vi "Smp_RAM_transfer.vi"(0 "Connection ID":T1, 5 "SaveFilePath":path caption="Temp file path", 9 "Read point":i32=1000, 11 "error in (no error)":errorcluster) -> (3 "Error Code":i16, 4 "Connection ID Out":T1, 6 "SaveFilePath.ref":path caption="Temp file path.ref", 10 "Stop":bool, 15 "error out":errorcluster)   [LabVIEW 2017]
uses:
  Driver/ConnectionID.ctl
  GL860_Driver.lvlib
panel:
  out "Progress bar":u8(slide) max=100 scale=0.0..100.0
  in  "Stop":bool
  # "Now transferring data..."
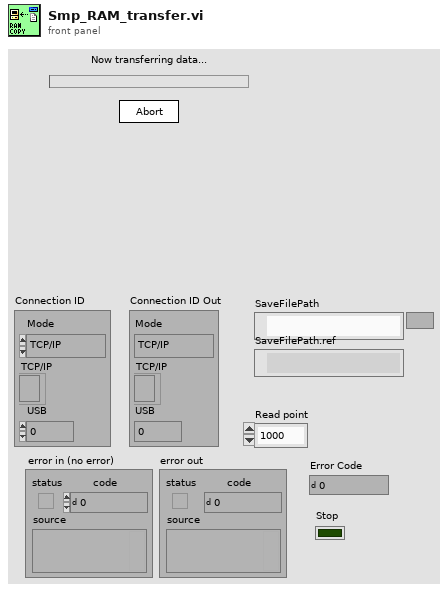
[diagram p1: front panel]
types:
  T1 = typedef "ConnectionID.ctl" = cluster{"Mode":enum16{"TCP/IP", "USB"}, "TCP/IP":refnum<k5>, "USB":i32}
  T2 = enum16{"open", "replace", "create", "open or create", "replace or create", "replace or create with confirmation"}
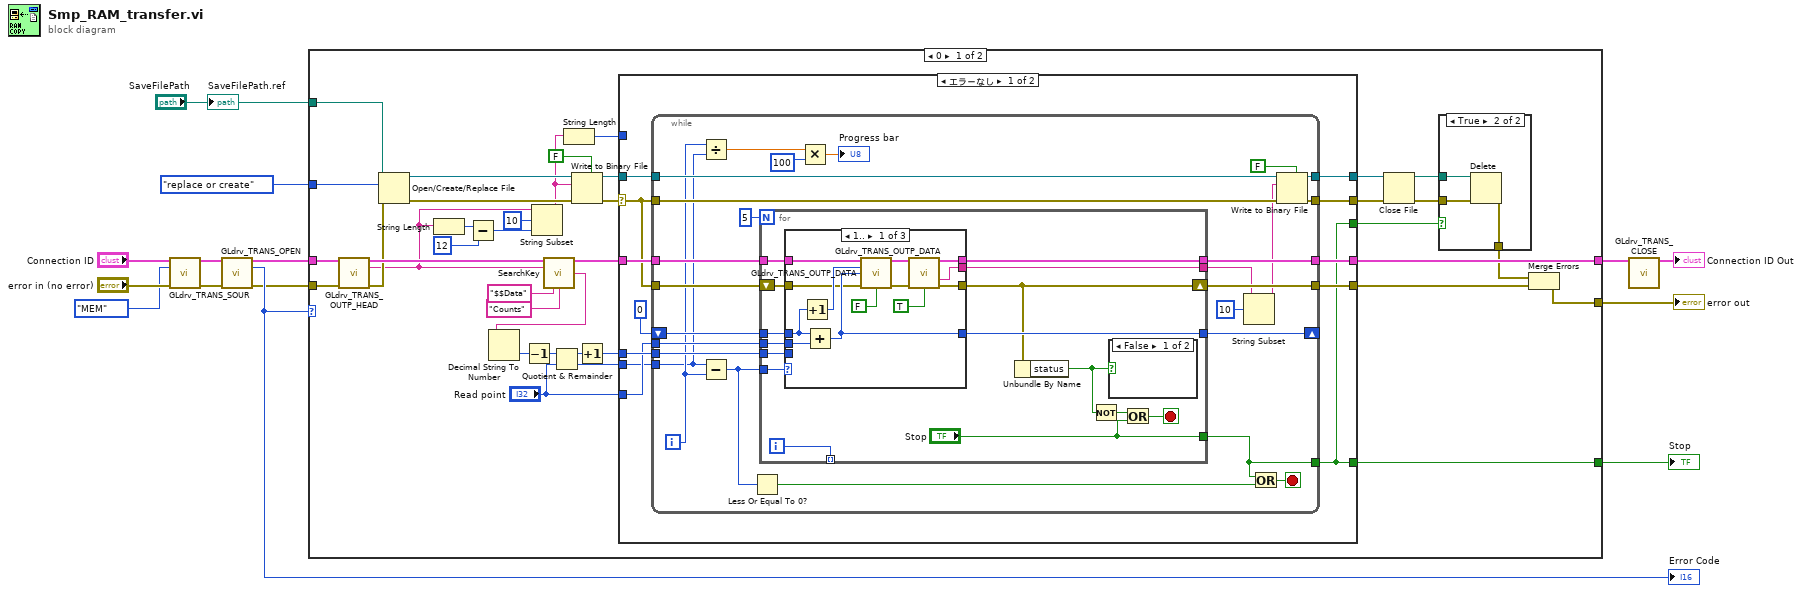
[diagram p0: block diagram]
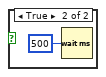
[diagram p3: hidden frame]
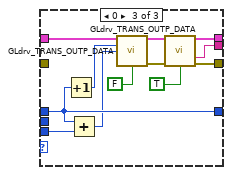
[diagram p5: hidden frame]
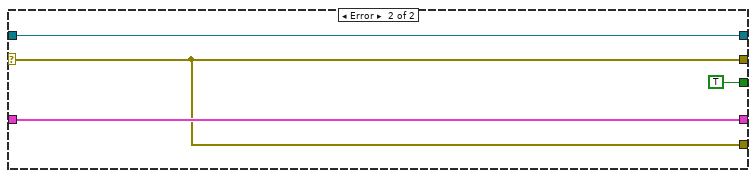
[diagram p6: hidden frame]
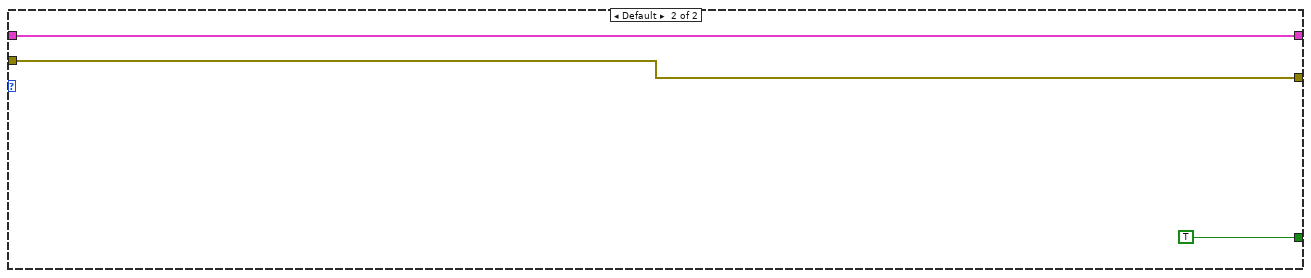
[diagram p7: hidden frame]
diagram:
  n1 = call "GLdrv_TRANS_SOUR.vi"("Connection ID"="Connection ID", "Mode"=enum16{"DISK", "MEM"}."MEM", "error in (no error)"="error in (no error)") -> ("Connection ID Out"=w8:T1, "error out"=w6:errorcluster)  [unwired: 9 in, 2 out]
  n2 = call "GLdrv_TRANS_OPEN.vi"("Connection ID"=w8, "error in (no error)"=w6) -> ("Connection ID Out"=w5:T1, "Error Code"=w7:i16, "error out"=w4:errorcluster)  [unwired: 10 in, 1 out]
  "Error Code" <- w7
  n3 = case shown="0" w7 {
    tunnel: [w50 w142] -> w3
    tunnel: [w48 w143] -> w1
    tunnel: [w43 TRUE ("Stop")] -> w14
    tunnel: "SaveFilePath" -> [w19 _]
    tunnel: T2."replace or create" ("operation (0:open)") -> [w40 _]
    tunnel: w5 -> [w39 w142]
    tunnel: w4 -> [w38 w143]
    frame 0 {
      n4 = call "GLdrv_TRANS_OUTP_HEAD.vi"("Connection ID"=w39, "error in (no error)"=w38) -> ("Connection ID Out"=w37:T1, "Data out"=w25:string, "error out"=w36:errorcluster)  [unwired: 11 in]
      n5 = Open/Create/Replace File(file path (use dialog)=w19, error in=w36, operation (0:open)=w40) -> (refnum out=w33:refnum<file>, error out=w34:errorcluster)  [unwired: 4 out]
      n6 = String Length(string=w25) -> (length=w24:i32)
      n7 = Subtract(x=w24, y=12) -> (x-y=w22:i32)
      n8 = String Subset(string=w25, offset (0)=10 ("オフセット（0）"), length (rest)=w22) -> (substring=w21:string)
      n9 = call "SearchKey.vi"("In"=w25, "KEY1"="$$Data", "KEY2"="Counts") -> ("String"=w27:string)  [unwired: 12 out]
      n10 = Decimal String To Number(string=w27) -> (number=w28:i32)  [unwired: 2 in, 1 out]
      n11 = Decrement(x=w28) -> (x-1=w42:i32)
      n12 = Quotient & Remainder(x=w42, y="Read point") -> (x-y*floor(x/y)=w45:i32, floor(x/y)=w44:i32)
      n13 = String Length(string=w21) -> (length=w20:i32)
      n14 = Write to Binary File(file (use dialog)=w33, data=w21, error in=w34, 5:FALSE ("prepend array or string size? (T)")) -> (refnum out=w32:refnum<file>, error out=w31:errorcluster)  [unwired: 3 out]
      n15 = Increment(x=w45) -> (x+1=w41:i32)
      n16 = case shown="エラーなし" w31 {
        selector: w31 -> [w61 w140]
        tunnel: w32 -> [w67 w139]
        tunnel: w37 -> [w66 w141]
        tunnel: w41 -> [w64 _]
        tunnel: w44 -> [w62 _]
        tunnel: "Read point" -> [w63 _]
        tunnel: [w60 w141] -> w50
        tunnel: [w59 w140] -> w49
        tunnel: [w58 w140] -> w47
        tunnel: [w57 w139] -> w46
        tunnel: [w56 _] -> w43
        tunnel: w20 -> [_ _]
        tunnel: [w56 TRUE ("Stop")] -> w17
        frame No Error {
          n17 = while {
            tunnel: w67 -> [w87]
            tunnel: w61 -> [w88]
            tunnel: w66 -> [w93]
            tunnel: w62 -> [w77]
            tunnel: [w92] -> w60
            tunnel: [w91] -> w59
            shift-right: [w89] -> _
            shift-left: 0 -> [w90]
            tunnel: w64 -> [w84]
            tunnel: [w86] -> w57
            tunnel: [w85] -> w58
            tunnel: w63 -> [w83]
            tunnel: w61 -> [w82]
            tunnel: [w72] -> w56
            i -> [w78]
            stop <- w79 stop-if-true
            n18 = Divide(x=w78, y=w77) -> (x/y=w74:dbl)
            n19 = Subtract(x=w77, y=w78) -> (x-y=w81:i32)
            n20 = Less Or Equal To 0?(x=w81) -> (x <= 0?=w80:bool)
            n21 = for {
              N: 5 -> [_]
              tunnel: w93 -> [w108]
              tunnel: [w107] -> w92
              tunnel: w90 -> [w106]
              tunnel: [w105] -> w89
              tunnel: [w96] -> w69
              tunnel: w84 -> [w104]
              tunnel: w83 -> [w103]
              tunnel: w81 -> [w101]
              tunnel: ["Stop"] -> w72
              shift-right: [w100] -> w91
              shift-left: w82 -> [w102]
              tunnel: [w95] -> _ mode=indexing
              i -> [w95]
              stop <- w98 stop-if-true
              n22 = case shown="1.." w101 {
                tunnel: w108 -> [w115 w125 w135]
                tunnel: [w117 w125 w133] -> w107
                tunnel: [w111 w124 w131] -> w100
                tunnel: w106 -> [w122 w123 w137]
                tunnel: [w113 w123 w137] -> w105
                tunnel: [w112 _ w132] -> w96
                tunnel: w104 -> [_ _ w136]
                tunnel: w103 -> [w121 _ _]
                tunnel: w102 -> [w110 w124 _]
                frame 1.. {
                  n23 = Increment(x=w122) -> (x+1=w114:i32)
                  n24 = Add(x=w122, y=w121) -> (x+y=w113:i32)
                  n25 = call "GLdrv_TRANS_OUTP_DATA.vi"("Connection ID"=w115, "Start Byte"=w114, "End Byte"=w113, "error in (no error)"=w110, "Query(f)"=FALSE) -> ("Connection ID Out"=w116:T1, "error out"=w120:errorcluster)  [unwired: 8 in, 1 out]
                  n26 = call "GLdrv_TRANS_OUTP_DATA.vi"("Connection ID"=w116, "error in (no error)"=w120, "Query(f)"=TRUE) -> ("Connection ID Out"=w117:T1, "Data out"=w112:string, "error out"=w111:errorcluster)  [unwired: 10 in]
                }
                frame ..-1 {
                }
                frame 0 {
                  n27 = Increment(x=w137) -> (x+1=w126:i32)
                  n28 = Add(x=w137, y=w136) -> (x+y=w127:i32)
                  n29 = call "GLdrv_TRANS_OUTP_DATA.vi"("Connection ID"=w135, "Start Byte"=w126, "End Byte"=w127, "Query(f)"=FALSE) -> ("Connection ID Out"=w134:T1, "error out"=w130:errorcluster)  [unwired: 9 in, 1 out]
                  n30 = call "GLdrv_TRANS_OUTP_DATA.vi"("Connection ID"=w134, "error in (no error)"=w130, "Query(f)"=TRUE) -> ("Connection ID Out"=w133:T1, "Data out"=w132:string, "error out"=w131:errorcluster)  [unwired: 10 in]
                }
              }
              n31 = Unbundle By Name(w100) -> ("status"=w94:bool)
              n32 = Not(x=w94) -> (.not. x?=w97:bool)
              n33 = case shown="FALSE" w94 {
                frame False {
                }
                frame True {
                  n34 = Wait (ms)(milliseconds to wait=u32 500) -> ()  [unwired: 1 out]
                }
              }
              n35 = Or(x=w97, y="Stop") -> (x .or. y?=w98:bool)
            }
            n36 = Multiply(x=w74, y=u8 100) -> (x*y=→"Progress bar":dbl)
            n37 = String Subset(string=w69, offset (0)=10 ("オフセット（0）")) -> (substring=w68:string)  [unwired: 1 in]
            n38 = Or(x=w72, y=w80) -> (x .or. y?=w79:bool)
            n39 = Write to Binary File(file (use dialog)=w87, data=w68, error in=w88, 5:FALSE ("prepend array or string size? (T)")) -> (refnum out=w86:refnum<file>, error out=w85:errorcluster)  [unwired: 3 out]
          }
        }
        frame Error {
        }
      }
      n40 = Close File(refnum=w46, error in=w47) -> (path=w18:path, error out=w16:errorcluster)
      n41 = case shown="TRUE" w17 {
        tunnel: w16 -> [w52 w55]
        tunnel: w18 -> [_ w53]
        tunnel: [w52 w54] -> w15
        frame False {
        }
        frame True {
          n42 = Delete(path (use dialog)=w53, error in=w55) -> (error out=w54:errorcluster)  [unwired: 5 out]
        }
      }
      n43 = Merge Errors(w15, w49) -> (w48:errorcluster)
    }
    frame Default {
    }
  }
  "error out" <- w1
  "Stop" <- w14
  n44 = call "GLdrv_TRANS_CLOSE.vi"("Connection ID"=w3) -> ("Connection ID Out"=→"Connection ID Out":T1)  [unwired: 12 in, 2 out]
  "SaveFilePath.ref" <- "SaveFilePath"
